vi "SOUR_POW_CORR_COLL_C_SEN_SEL.vi"(0 "VISA IN":refnum<visa-resource-name>="GPIB1::16::INSTR", 1 "Power Meter Channel":string(combo)="A", 5 "error in":errorcluster, 7 "Channel":i32=1) -> (14 "VISA Out":refnum<visa-resource-name>, 19 "error out":errorcluster)   [LabVIEW 2018, in "PNA-X.lvlib"]
doc: "SOURce<cnum>:POWer:CORRection:COLLect:<pmChan>SENsor:SELect \n(Read-Write) Sets and returns the power sensor channel (A or B) to be used. This performs the same \nfunction as the Use this sensor only checkbox in the Power Sensor Settings dialog. \nNote: This write portion of this command is only necessary when performing an SMC calibration. \nParameters \n<cnum> Any existing channel number. If unspecified, value is set to 1 \n<pmChan> Power Meter channel. Choose from: \nA - Channel A \nB - Channel B \nExamples SOUR:POW:CORR:COLL:<pmChan>SEN:SEL 'Write \nsource1:power2:correction:collect:bsensor:select? 1e9 'Read \nQuery Syntax SOURce:POWer:CORRection:COLLect:ASENsor:SELect? <Frequency> \nSOURce:POWer:CORRection:COLLect:BSENsor:SELect? <Frequency> \nReturns a boolean 1 or 0 (true or false) indicating whether the sensor is to be \nused at the specified frequency. \nIf frequency checking is OFF, then the <Frequency> parameter is ignored. The \nquery returns if the sensor is selected for ALL frequencies. \nReturn Type Numeric \nDefault Not Applicable"
uses:
  PNA-X.lvlib
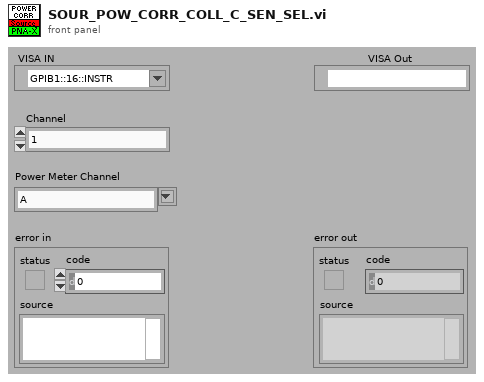
[diagram p1: front panel]
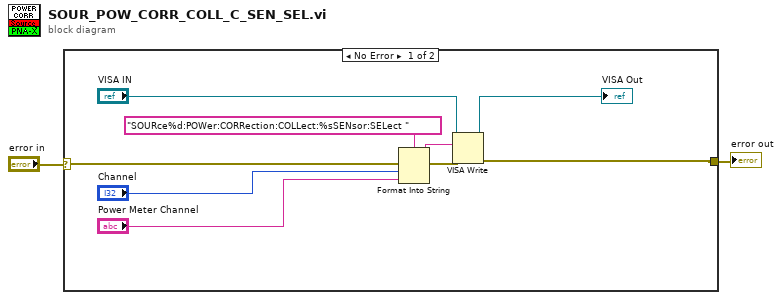
[diagram p0: block diagram]
diagram:
  n1 = case shown="No Error" "error in" {
    selector: "error in" -> [w11 w12]
    tunnel: [w6 w12] -> w1
    frame No Error {
      n2 = Format Into String(format string="SOURce%d:POWer:CORRection:COLLect:%sSENsor:SELect " ("Cmdline"), error in=w11, "Channel", "Power Meter Channel") -> (resulting string=w9:string, error out=w10:errorcluster)  [unwired: 1 in]
      n3 = VISA Write(VISA resource name="VISA IN", write buffer=w9, error in (no error)=w10) -> (VISA resource name out=→"VISA Out":refnum<visa-resource-name>, error out=w6:errorcluster)  [unwired: 1 out]
    }
    frame Error {
    }
  }
  "error out" <- w1
